vi "SPI API Dynamic FPGA Main.vi"() -> ()   [LabVIEW 2014]
uses:
  <vilib>/NI/LVFPGA Adv Session Resources/ResourceInfo.ctl
  <userlib>/_OpenG.lib/lvdata/lvdata.llb/Type Descriptor Header__ogtk.ctl
  <userlib>/_OpenG.lib/lvdata/lvdata.llb/Type Descriptor Enumeration__ogtk.ctl
  Source/Shared/MCP23S17/Chip Address.ctl
  <vilib>/Utility/VariantDataType/Type.ctl
  <vilib>/NI/LVFPGA Adv Session Resources/OpenByNameSubVI.vi
  <vilib>/FPGAPlugInAG/Dynamic/niLvFpga_Reset_Dynamic.vi
  <vilib>/FPGAPlugInAG/Dynamic/niLvFpga_Run_Dynamic.vi
  <vilib>/rvi/interface/common/dynamic/niFpgaEscapeDelimiterAndNull.vi
  <vilib>/Utility/error.llb/Error Cluster From Error Code.vi
  <vilib>/rvi/errors/niLvFpgaAdjustHostInterfaceError.vi
  Source/Shared/MCP23S17/Update Mode All Pins.vi
  Source/Shared/MCP23S17/Write Digital All Pins.vi
  <vilib>/FPGAPlugInAG/Dynamic/niLvFpga_Close_Dynamic.vi
  <vilib>/rvi/interface/nirviMethod/nirviMethod.xnode
  <vilib>/NI/LVFPGA Adv Session Resources/OpenByName.xnode
  <vilib>/rvi/interface/nirviReadWriteControl/nirviReadWriteControl.xnode
  <vilib>/rvi/interface/nirviCloseFPGA/nirviCloseFPGA.xnode
  Source/Shared/SLSC configuration Shared.lvlib
  <vilib>/NI/LVFPGA Adv Session Resources/LVFPGAAdvSessionResources.lvlib
  NiFpgaLv.dll
  <vilib>/rvi/interface/Simulation/niFpgaSimulationCallBeginRW.vi
  <vilib>/FPGAPlugInAG/Dynamic/niLvFpga_WriteFifo_Dynamic.vi
  <vilib>/rvi/errors/niLvFpgaMergeErrorWithErrorCode.vi
  <vilib>/Utility/VariantDataType/VariantType.lvlib
panel:
  out "Array 3":string[](array[string])
  out "Array 2":T1[](array[typedef]) {"type" format="%.0x"}
  out "Type Descriptor":i16[][](array[numeric])
  out "Resource info out":T3[](array[typedef])
  in  "Value":u16 format="%016b"
  in  "Boolean":bool
  out "Array":u64[](array[numeric])
  out "SPI Command":u32 format="%.0b"
  out "Transfer Length (bits)":u8
  in  "Chip Select":u8
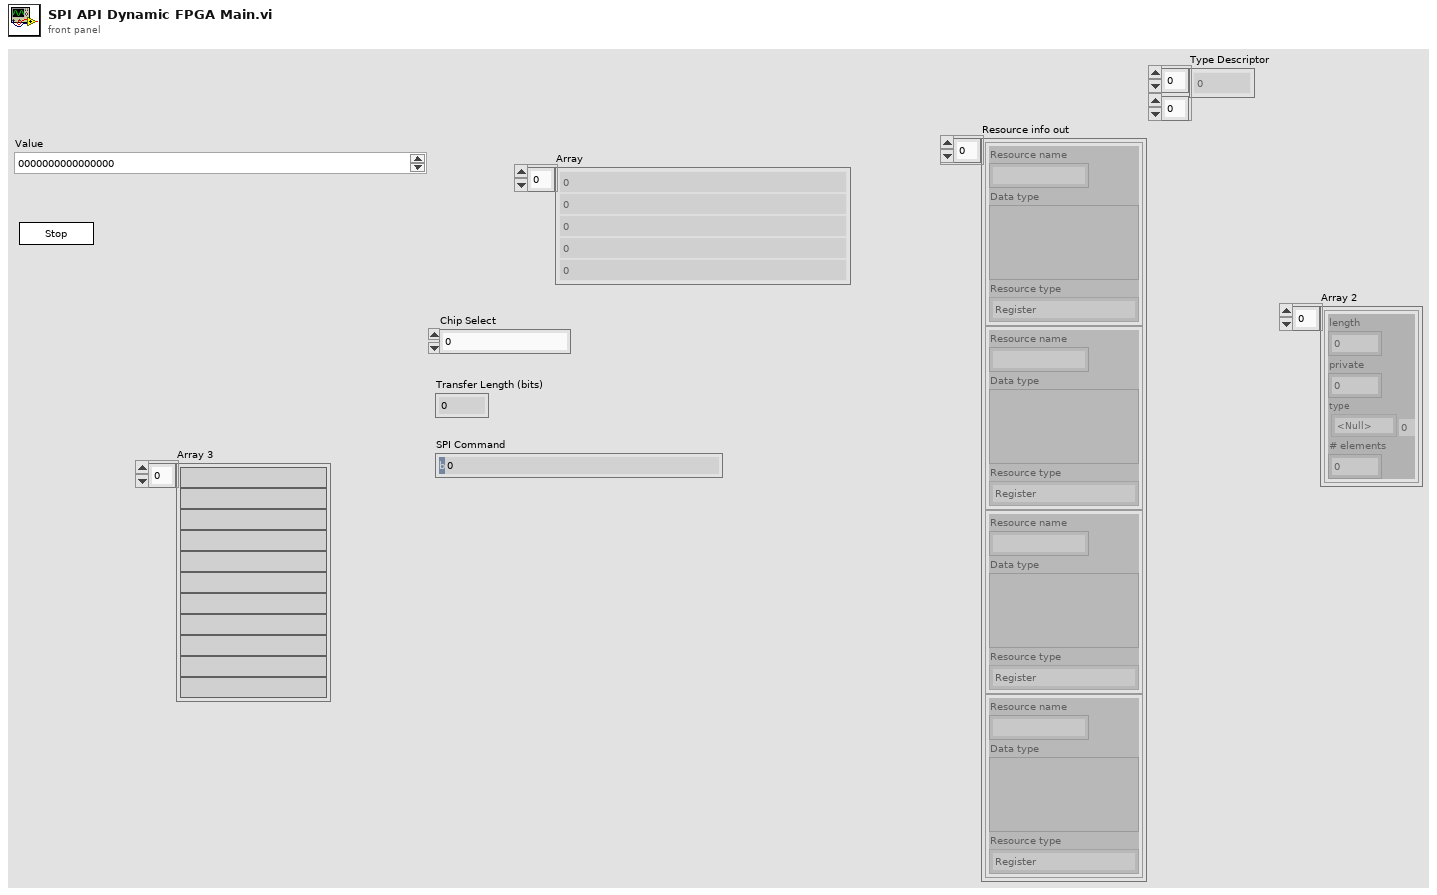
[diagram p1: front panel]
types:
  T1 = typedef "Type Descriptor Header__ogtk.ctl" = cluster{"length":u16, "private":u8, "type":T2, "# elements":u16}
  T2 = typedef "Type Descriptor Enumeration__ogtk.ctl" = enum8{"<Null>", "I8", "I16", "I32", "I64", "U8", "U16", "U32", "U64", "SGL", "DBL", "EXT", "CSG", "CDB", "CXT", "0x0F", "0x10", "0x11", "0x12", "0x13", "0x14", "Enum U8", "Enum U16", "Enum U32", "Enum U64", "SGL PQ", "DBL PQ", "EXT PQ", "CSG PQ", "CDB PQ", "CXT PQ", "0x1F", "0x20", "Boolean", "0x22", "0x23", "0x24", "0x25", "0x26", "0x27", "0x28", "0x29", "0x2A", "0x2B", "0x2C", "0x2D", "0x2E", "0x2F", "String", "0x31", "Path", "Pict", "0x34", "0x35", "0x36", "DAQ", "0x38", "0x39", "0x3A", "0x3B", "0x3C", "0x3D", "0x3E", "0x3F", "Array", "0x41", "0x42", "0x43", "0x44", "0x45", "0x46", "0x47", "0x48", "0x49", "0x4A", "0x4B", "0x4C", "0x4D", "0x4E", "0x4F", "Cluster", "0x51", "0x52", "Variant", "Waveform", "0x55", "0x56", "0x57", "0x58", "0x59", "0x5A", "0x5B", "0x5C", "0x5D", "0x5E", "0x5F", "0x60", "0x61", "0x62", "0x63", "0x64", "0x65", "0x66", "0x67", "0x68", "0x69", "0x6A", "0x6B", "0x6C", "0x6D", "0x6E", "0x6F", "Refnum"}
  T3 = typedef "LVFPGAAdvSessionResources.lvlib/ResourceInfo.ctl" = cluster{"Resource name":string, "Data type":variant, "Resource type":enum16{"Register", "Host To Target FIFO", "Target To Host FIFO"}}
  T4 = cluster{"Divide Value":u8, "Transfer Length (bits)":u8, "CS Asserted Polarity":bool, "Clock Polarity (CPOL)":bool, "Clock Phase (CPHA)":bool, "Lengthen MISO Setup":bool, "Direction Change Bit":u8, "MOSI Starts as Output":bool, "Tristatable MOSI":bool}
  T5 = typedef "SLSC configuration Shared.lvlib/Chip Address.ctl" = u8
  T6 = typedef "VariantType.lvlib/Type.ctl" = enum8{"Invalid Type", "Void", "I8", "I16", "I32", "I64", "U8", "U16", "U32", "U64", "Single Float", "Double Float", "Extended Float", "Single Complex", "Double Complex", "Extended Complex", "Enum U8", "Enum U16", "Enum U32", "Enum U64", "Single Float With Unit", "Double Float With Unit", "Extended Float With Unit", "Single Complex with Unit", "Double Complex with Unit", "Extended Complex with Unit", "Boolean", "String", "Path", "Picture", "Tag", "Array", "Cluster", "Variant", "LV Variant", "Waveform", "Timestamp", "Digital Waveform", "Digital Data", "ExpressData", "Refnum", "External Data", "VI", "Poly VI", "LabVIEW Class Instance", "Fixed Point"}
  T7 = enum16{"Register", "Host To Target FIFO", "Target To Host FIFO"}
  T8 = typedef "Type Descriptor__ogtk.ctl" = i16[]
  T9 = typedef "SLSC configuration Shared.lvlib/SPI Command.ctl" = cluster{"SPI Command":u32, "Transfer Length":u8}
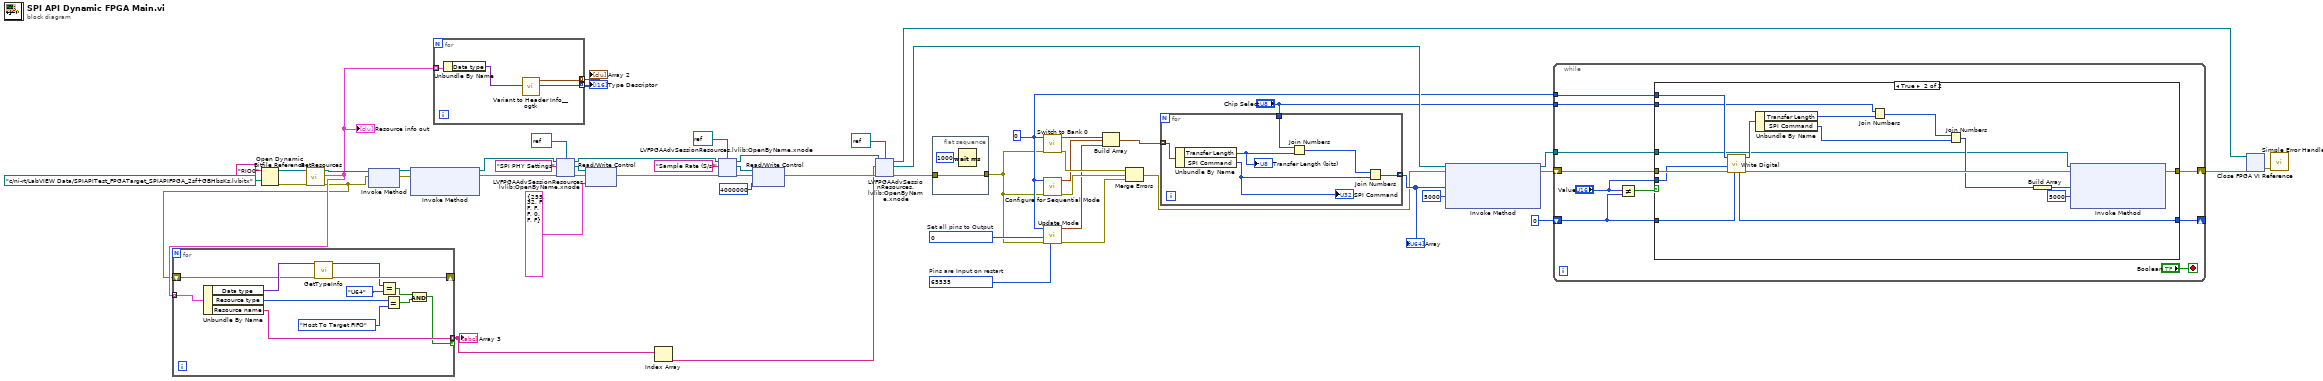
[diagram p0: block diagram]
diagram:
  w15 = T5 0 ("Chip Address (A2 A1 A0)")
  w49 = u16 0  # Set all pins to Output
  w50 = u16 65535  # Pins are Input on restart
  n1 = Open Dynamic Bitfile Reference(0:"RIO0" ("Device address"), 1:path "c:/ni-rt/LabVIEW Data/SPIAPITest_FPGATarget_SPIAPIFPGA_2sf+GBHbsKs.lvbitx" ("Bitfile path")) -> (5:w8:refnum<k20>, 8:w9:errorcluster)  [unwired: 3 in]
  n2 = call <vilib>:"GetResources.vi"("error in (no error)"=w9, "FPGA VI Reference in"=w8) -> ("error out"=w3:errorcluster, "Resource info out"=w4:T3[], "FPGA VI Reference out"=w7:refnum<k20>)  [unwired: 7 in]
  "Resource info out" <- w4
  n3 = for {
    tunnel: w4 -> [w65] mode=indexing
    shift-right: [w60] -> _
    shift-left: w3 -> [w61]
    tunnel: [w55] -> w2 mode=indexing if=w54
    n4 = Unbundle By Name(w65) -> ("Data type"=w62:variant, "Resource type"=w64:T7, "Resource name"=w55:string)
    n5 = call <vilib>:"GetTypeInfo.vi"("error in (no error)"=w61, "Variant"=w62) -> ("error out"=w60:errorcluster, "Type Enum"=w58:T6)  [unwired: 5 in, 3 out]
    n6 = Equal?(x=w58, y=Type."U64" ("Type Enum")) -> (x = y?=w57:bool)
    n7 = Equal?(x=w64, y=T7."Host To Target FIFO" ("Resource type")) -> (x = y?=w56:bool)
    n8 = And(x=w57, y=w56) -> (x .and. y?=w54:bool)
  }
  "Array 3" <- w2
  n9 = xnode "Invoke Method"("FPGA VI Reference In"=w7, "error in"=w3) -> ("FPGA VI Reference Out"=w34:refnum<k20>, "error out"=w35:errorcluster)
  n10 = xnode "Invoke Method"("FPGA VI Reference In"=w34, "error in"=w35) -> ("FPGA VI Reference Out"=w32:refnum<k20>, "error out"=w31:errorcluster)  [unwired: 1 in]
  n11 = for {
    tunnel: w4 -> [w69] mode=indexing
    tunnel: [w67] -> w6 mode=indexing
    tunnel: [w66] -> w5 mode=indexing
    n12 = Unbundle By Name(w69) -> ("Data type"=w68:variant)
    n13 = call <userlib>:"Variant to Header Info__ogtk.vi"("Variant"=w68) -> ("Type Descriptor Header"=w66:T1, "Type Descriptor"=w67:T8)  [unwired: 3 in, 1 out]
  }
  "Type Descriptor" <- w6
  "Array 2" <- w5
  n14 = xnode "LVFPGAAdvSessionResources.lvlib:OpenByName.xnode"("FPGA VI Reference in"=w32, "Resource name in"="SPI PHY Settings", "Single resource reference type in"=refnum<k20> refnum, "Error in"=w31) -> ("Single resource reference out"=w30:refnum<k20>, "Error out"=w29:errorcluster, "FPGA VI Reference out"=w26:refnum<k20>)
  n15 = xnode "Read/Write Control"("FPGA VI Reference In"=w30, "error in"=w29, "Value"=T4 {"Divide Value"=255, "Transfer Length (bits)"=32, "CS Asserted Polarity"=FALSE, "Clock Polarity (CPOL)"=FALSE, "Clock Phase (CPHA)"=FALSE, "Lengthen MISO Setup"=FALSE, "Direction Change Bit"=0, "MOSI Starts as Output"=FALSE, "Tristatable MOSI"=FALSE} ("SPI PHY Settings")) -> ("error out"=w27:errorcluster)  [unwired: 1 out]
  n16 = Index Array(array=w2) -> (element=w1:string)  [unwired: 1 in]
  n17 = xnode "LVFPGAAdvSessionResources.lvlib:OpenByName.xnode"("FPGA VI Reference in"=w26, "Resource name in"="Sample Rate (S/s)", "Single resource reference type in"=refnum<k20> refnum, "Error in"=w27) -> ("Single resource reference out"=w23:refnum<k20>, "Error out"=w24:errorcluster, "FPGA VI Reference out"=w20:refnum<k20>)
  n18 = xnode "Read/Write Control"("FPGA VI Reference In"=w23, "error in"=w24, "Value"=u32 4000000 ("Sample Rate (S/s)")) -> ("error out"=w21:errorcluster)  [unwired: 1 out]
  n19 = xnode "LVFPGAAdvSessionResources.lvlib:OpenByName.xnode"("FPGA VI Reference in"=w20, "Resource name in"=w1, "Single resource reference type in"=refnum<k20> refnum, "Error in"=w21) -> ("Single resource reference out"=w51:refnum<k20>, "Error out"=w12:errorcluster, "FPGA VI Reference out"=w36:refnum<k20>)
  n20 = flat-sequence {
    tunnel: w12 -> [w70]
    tunnel: [w70] -> w11
    frame #0 {
      n21 = Wait (ms)(milliseconds to wait=u32 1000) -> ()  [unwired: 1 out]
    }
  }
  n22 = call "Switch to Bank 0.vi"("error in (no error)"=w11, "Chip Address (A2 A1 A0)"=w15) -> ("error out"=w48:errorcluster, "SPI Command"=w45:T9)  [unwired: 8 in]
  n23 = call "Configure for Sequential Mode.vi"("error in (no error)"=w11, "Chip Address (A2 A1 A0)"=w15) -> ("error out"=w47:errorcluster, "SPI Command"=w44:T9)  [unwired: 8 in]
  n24 = call-poly "Update Mode.vi"("Mode Cache in"=w50, "error in (no error)"=w11, "Mode"=w49, "Chip Address (A2 A1 A0)"=w15) -> ("error out"=w46:errorcluster, "SPI Command"=w43:T9)  [unwired: 5 in, 1 out]
  n25 = Build Array(w45, w44, w43) -> (w42:T9[])
  n26 = Merge Errors(w48, w47, w46) -> (w39:errorcluster)
  n27 = for {
    tunnel: w42 -> [w74] mode=indexing
    tunnel: [w73] -> w41 mode=indexing
    tunnel: "Chip Select" -> [w72]
    n28 = Unbundle By Name(w74) -> ("Transfer Length"=w76:u8, "SPI Command"=w77:u32)
    "Transfer Length (bits)" <- w76
    "SPI Command" <- w77
    n29 = Join Numbers(hi=w72, lo=w76) -> ((hi.lo)=w75:u16)
    n30 = Join Numbers(hi=w75, lo=w77) -> ((hi.lo)=w73:u64)
  }
  "Array" <- w41
  n31 = xnode "Invoke Method"("FPGA VI Reference In"=w51, "error in"=w39, "Data"=w41, "Timeout (ms)"=5000) -> ("FPGA VI Reference Out"=w14:refnum<k20>, "error out"=w17:errorcluster)  [unwired: 1 out]
  n32 = while {
    shift-right: [w83] -> w16
    shift-left: w17 -> [w86]
    tunnel: w15 -> [w85]
    tunnel: w14 -> [w82]
    tunnel: "Chip Select" -> [w81]
    shift-right: [w80] -> _
    shift-left: u16 0 ("Output Cache in") -> [w79]
    stop <- "Boolean" stop-if-true
    n33 = Not Equal?(x="Value", y=w79) -> (x != y?=w84:bool)
    n34 = case shown="True" w84 {
      tunnel: w86 -> [w89 w105]
      tunnel: w85 -> [_ w104]
      tunnel: [w89 w95] -> w83
      tunnel: w82 -> [_ w94]
      tunnel: w81 -> [_ w93]
      tunnel: w79 -> [w88 w91]
      tunnel: [w88 w90] -> w80
      tunnel: "Value" -> [_ w92]
      frame False {
      }
      frame True {
        n35 = call-poly "Write Digital.vi"("Output Cache in"=w91, "error in (no error)"=w105, "Value"=w92, "Chip Address (A2 A1 A0)"=w104) -> ("error out"=w103:errorcluster, "SPI Command"=w99:T9, "Output Cache out"=w90:u16)  [unwired: 5 in]
        n36 = Unbundle By Name(w99) -> ("Transfer Length"=w101:u8, "SPI Command"=w102:u32)
        n37 = Join Numbers(hi=w93, lo=w101) -> ((hi.lo)=w100:u16)
        n38 = Join Numbers(hi=w100, lo=w102) -> ((hi.lo)=w98:u64)
        n39 = Build Array(w98) -> (w97:u64[])
        n40 = xnode "Invoke Method"("FPGA VI Reference In"=w94, "error in"=w103, "Data"=w97, "Timeout (ms)"=5000) -> ("error out"=w95:errorcluster)  [unwired: 2 out]
      }
    }
  }
  n41 = xnode "Close FPGA VI Reference"("FPGA VI Reference In"=w36, "error in"=w16) -> ("error out"=w38:errorcluster)
  n42 = call <vilib>:"Simple Error Handler.vi"("error in (no error)"=w38) -> ()  [unwired: 1 in, 8 out]
